vi "FTW-Collection-Construct-KeyValuePairs.vi"(5 "Key-Value Pairs":T1[](array[typedef]), 11 "error in":errorcluster) -> (4 "Collection":refnum<class "FTW-Collection.lvclass">, 15 "error out":errorcluster)   [LabVIEW 2013, in "FTW-Collection.lvclass"]
uses:
  FTW-Collection.lvclass
  FTW-Collection-KeyValuePair.ctl
panel:
  # "Inputs"
  # "Outputs"
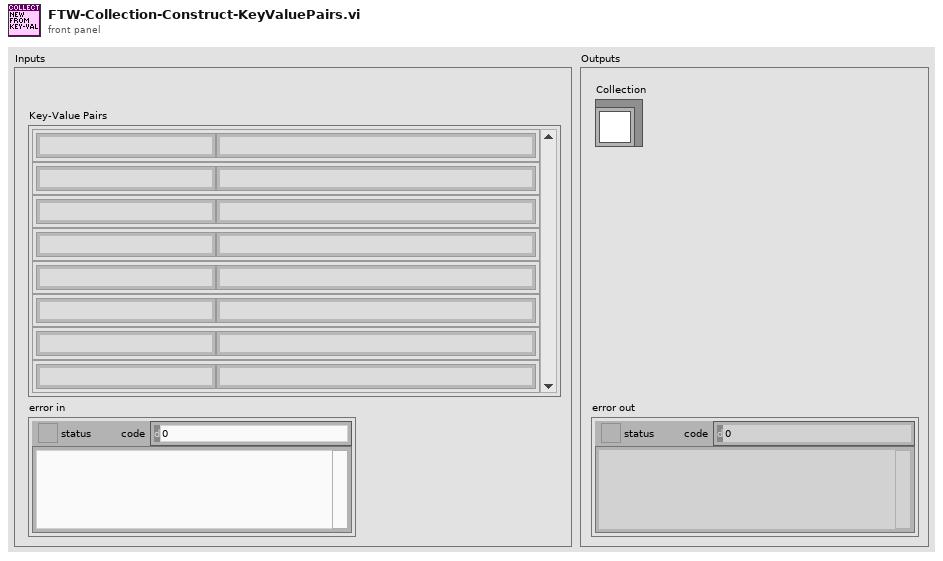
[diagram p1: front panel]
types:
  T1 = typedef "FTW-Collection-KeyValuePair.ctl" = cluster{"Key":string, "Value":string}
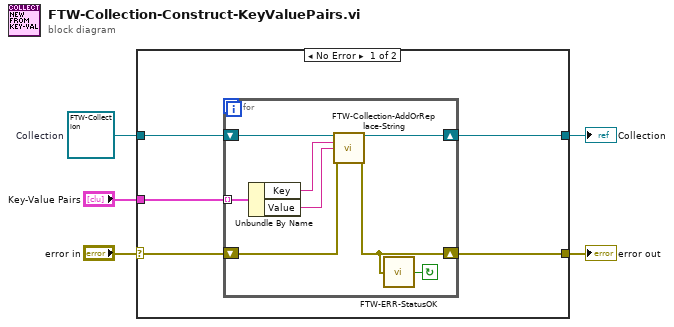
[diagram p0: block diagram]
diagram:
  w2 = refnum<class "FTW-Collection.lvclass"> refnum  # Collection
  n1 = case shown="No Error" "error in" {
    selector: "error in" -> [w9 w19]
    tunnel: [w8 w19] -> w5
    tunnel: [w10 _] -> w3
    tunnel: w2 -> [w7 _]
    tunnel: "Key-Value Pairs" -> [w6 _]
    frame No Error {
      n2 = for {
        shift-right: [w18] -> w10
        shift-left: w7 -> [w16]
        shift-right: [w12] -> w8
        shift-left: w9 -> [w17]
        tunnel: w6 -> [w15] mode=indexing
        stop <- w11 continue-if-true
        n3 = Unbundle By Name(w15) -> ("Key"=w14:string, "Value"=w13:string)
        n4 = call "FTW-Collection-AddOrReplace-String.vi"("Collection"=w16, "Key"=w14, "Value"=w13, "error in"=w17) -> ("Collection out"=w18:refnum<class "FTW-Collection.lvclass">, "error out"=w12:errorcluster)  [unwired: 9 in, 1 out]
        n5 = call "FTW-ERR-StatusOK.vi"("error to check"=w12) -> ("Status OK?"=w11:bool)
      }
    }
    frame Error {
    }
  }
  "error out" <- w5
  "Collection" <- w3
